vi "Set Operation Mode.vi"(8 "error in (no error)":errorcluster, 10 "Operating Modes":T1, 11 "VISA session":refnum<visa-resource-name>) -> (0 "error out":errorcluster, 3 "dup VISA session":refnum<visa-resource-name>)   [LabVIEW 2011, in "Magna PSU.lvlib"]
doc: "This VI form enables or disables the front start, stop, arm, and clear keys."
uses:
  Magna PSU.lvlib
  Operating Modes Enum.ctl
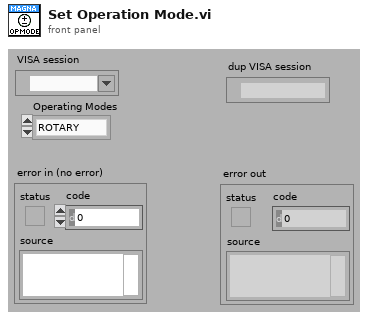
[diagram p1: front panel]
types:
  T1 = typedef "Magna PSU.lvlib/Operating Modes Enum.ctl" = enum16{"ROTARY", "KEYPAD", "EXT PGM", "REMOTE"}
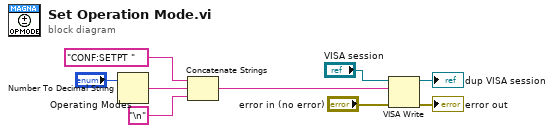
[diagram p0: block diagram]
diagram:
  n1 = Number To Decimal String(number="Operating Modes") -> (decimal integer string=w1:string)  [unwired: 1 in]
  n2 = Concatenate Strings("CONF:SETPT ", w1, "\n") -> (w8:string)
  n3 = VISA Write(VISA resource name="VISA session", write buffer=w8, error in (no error)="error in (no error)") -> (VISA resource name out=→"dup VISA session":refnum<visa-resource-name>, error out=→"error out":errorcluster)  [unwired: 1 out]
